vi "Status Run.vi"(8 "error in":errorcluster, 9 "Finished Late? [i-1]":bool, 10 "Iteration Duration":i64, 11 "RT Data In":T1 {"Compiled Data"."9759 RevB"."Settings"."ControlCals"."ThetaLH (deg)" format="%.3f"; "Compiled Data"."9759 RevB"."Settings"."ControlCals"."ULHLag (sec)" format="%.3f"; "Compiled Data"."9759 RevB"."Settings"."ControlCals"."USLag (sec)" format="%.3f"; "Compiled Data"."9759 RevB"."Settings"."ControlCals"."TLead (sec)" format="%.3f"; "Compiled Data"."9759 RevB"."Settings"."ControlCals"."TLag (sec)" format="%.3f"}) -> (0 "error out":errorcluster, 2 "Stop":bool, 3 "RT Data Out":T1 {"Compiled Data"."9759 RevB"."Settings"."ControlCals"."ThetaLH (deg)" format="%.3f"; "Compiled Data"."9759 RevB"."Settings"."ControlCals"."ULHLag (sec)" format="%.3f"; "Compiled Data"."9759 RevB"."Settings"."ControlCals"."USLag (sec)" format="%.3f"; "Compiled Data"."9759 RevB"."Settings"."ControlCals"."TLead (sec)" format="%.3f"; "Compiled Data"."9759 RevB"."Settings"."ControlCals"."TLag (sec)" format="%.3f"})   [LabVIEW 2015, in "NI 9759 RevB Custom Device.lvlib"]
uses:
  NI 9759 RevB Custom Device.lvlib
  Shared/Types/RT Data.ctl
  Shared/Types/Compiled Data.ctl
  Shared/Types/RT Init Data.ctl
  Shared/Types/RT Status.ctl
  Shared/Types/9759 RevB.ctl
  Shared/Types/FPGA Refs.ctl
  Shared/Types/Generic FPGA Ref.ctl
  Shared/Types/9759 RevB FPGA Ref.ctl
  <vilib>/NI Veristand/Custom Device Tools/Custom Device Utility Library/Custom Device Utility Library.lvlib
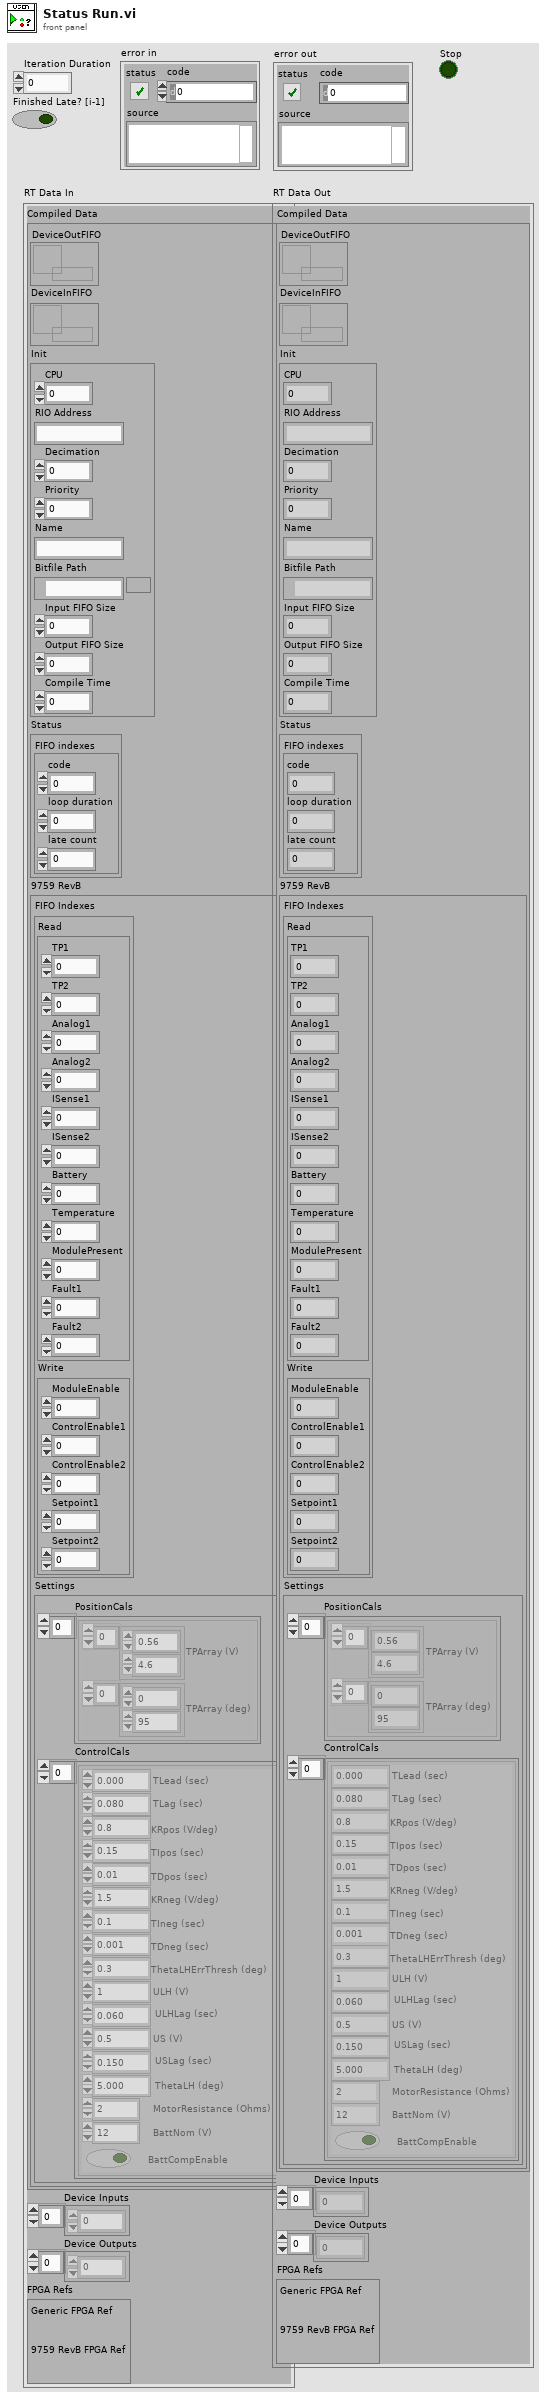
[diagram p1: front panel]
types:
  T1 = typedef "NI 9759 RevB Custom Device.lvlib/RT Data.ctl" = cluster{"Compiled Data":T2, "Device Inputs":dbl[], "Device Outputs":dbl[], "FPGA Refs":T6}
  T2 = typedef "NI 9759 RevB Custom Device.lvlib/Compiled Data.ctl" = cluster{"DeviceOutFIFO":refnum<k33>, "DeviceInFIFO":refnum<k33>, "Init":T3, "Status":T4, "9759 RevB":T5}
  T3 = typedef "NI 9759 RevB Custom Device.lvlib/RT Init Data.ctl" = cluster{"CPU":i32, "RIO Address":string, "Decimation":i32, "Priority":i32, "Name":string, "Bitfile Path":path, "Input FIFO Size":i32, "Output FIFO Size":i32, "Compile Time":dbl}
  T4 = typedef "NI 9759 RevB Custom Device.lvlib/RT Status.ctl" = cluster{"FIFO indexes":cluster{"code":i32, "loop duration":i32, "late count":i32}}
  T5 = typedef "NI 9759 RevB Custom Device.lvlib/9759 RevB.ctl" = cluster{"FIFO Indexes":cluster{"Read":cluster{"TP1":i32, "TP2":i32, "Analog1":i32, "Analog2":i32, "ISense1":i32, "ISense2":i32, "Battery":i32, "Temperature":i32, "ModulePresent":i32, "Fault1":i32, "Fault2":i32}, "Write":cluster{"ModuleEnable":i32, "ControlEnable1":i32, "ControlEnable2":i32, "Setpoint1":i32, "Setpoint2":i32}}, "Settings":cluster{"PositionCals":cluster{"TPArray (V)":sgl[], "TPArray (deg)":sgl[]}[], "ControlCals":cluster{"TLead (sec)":sgl, "TLag (sec)":sgl, "KRpos (V/deg)":sgl, "TIpos (sec)":sgl, "TDpos (sec)":sgl, "KRneg (V/deg)":sgl, "TIneg (sec)":sgl, "TDneg (sec)":sgl, "ThetaLHErrThresh (deg)":sgl, "ULH (V)":sgl, "ULHLag (sec)":sgl, "US (V)":sgl, "USLag (sec)":sgl, "ThetaLH (deg)":sgl, "MotorResistance (Ohms)":sgl, "BattNom (V)":sgl, "BattCompEnable":bool}[]}}
  T6 = typedef "NI 9759 RevB Custom Device.lvlib/FPGA Refs.ctl" = cluster{"Generic FPGA Ref":T7, "9759 RevB FPGA Ref":T8}
  T7 = typedef "NI 9759 RevB Custom Device.lvlib/Generic FPGA Ref.ctl" = refnum<k20>
  T8 = typedef "NI 9759 RevB Custom Device.lvlib/9759 RevB FPGA Ref.ctl" = refnum<k20>
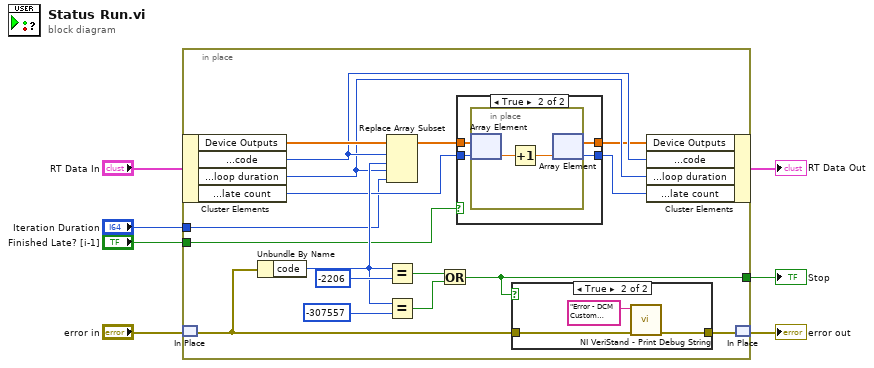
[diagram p0: block diagram]
diagram:
  n1 = in-place {
    in-place-border: "Iteration Duration" -> [w11]
    in-place-border: "Finished Late? [i-1]" -> [w12]
    in-place-border: [w10] -> w7
    n2 = in-place-cluster #1("RT Data In") -> ("Device Outputs"=w19:dbl[], "Compiled Data.Status.FIFO indexes.code"=w18:i32, "Compiled Data.Status.FIFO indexes.loop duration"=w17:i32, "Compiled Data.Status.FIFO indexes.late count"=w15:i32)
    n3 = in-place-match #2("error in") -> (w9:errorcluster)
    n4 = Unbundle By Name(w9) -> ("code"=w23:i32)
    n5 = Replace Array Subset(array=w19, new element #1=w23, index #1=w18, new element #2=w11, index #2=w17) -> (w16:dbl[])
    n6 = Equal?(x=w23, y=-2206) -> (x = y?=w21:bool)
    n7 = Equal?(x=w23, y=-307557) -> (x = y?=w20:bool)
    n8 = Or(x=w21, y=w20) -> (x .or. y?=w10:bool)
    n9 = case shown="True" w12 {
      tunnel: w16 -> [w30 w34]
      tunnel: w15 -> [w29 w33]
      tunnel: [w29 w32] -> w14
      tunnel: [w30 w31] -> w13
      frame False {
      }
      frame True {
        n10 = in-place {
          n11 = in-place-array #3(w34, w33) -> (w36:dbl)
          n12 = Increment(x=w36) -> (x+1=w35:dbl)
          n13 = in-place-array #3(w35) -> (w31:dbl[], w32:i32)
        }
      }
    }
    n14 = case shown="True" w10 {
      tunnel: w9 -> [w25 w27]
      tunnel: [w25 w26] -> w8
      frame False {
      }
      frame True {
        n15 = call <vilib>:"NI VeriStand - Print Debug String.vi"("error in (no error)"=w27, "Message"="Error - DCM Custom Device is shutting down\n") -> ("error out"=w26:errorcluster)  [unwired: 9 in]
      }
    }
    n16 = in-place-cluster #1("Device Outputs"=w13, "Compiled Data.Status.FIFO indexes.code"=w18, "Compiled Data.Status.FIFO indexes.loop duration"=w17, "Compiled Data.Status.FIFO indexes.late count"=w14) -> (→"RT Data Out":T1)
    n17 = in-place-match #2(w8) -> (→"error out":errorcluster)
  }
  "Stop" <- w7
